vi "OpenVisualizations.vi"(8 "ErrorArray in":errorcluster[](array[cluster]), 11 "Visualization VI Paths":path[](array[path])) -> (0 "ErrorArray out":errorcluster[](array[cluster]))   [LabVIEW 2018]
uses:
  VisulaizationManagement/VisualizationManagerActions.ctl
  VisulaizationManagement/OpenVisualizationVIs.ctl
  <userlib>/NIST/NISTErrorLib/NISTErrorLib.lvlib
  NistPluggableModules/TestClass/Test.lvclass
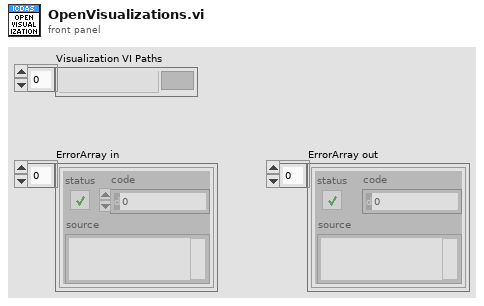
[diagram p1: front panel]
types:
  T1 = typedef "VisualizationManagerActions.ctl" = enum16{"Set", "LoadModVI", "PopOutModVI"}
  T2 = typedef "OpenVisualizationVIs.ctl" = cluster{"Module Name":string, "VI ref":refnum<vi>, "In SubPanel?":bool}
  T3 = typedef "cntlRefs.ctl" = cluster{"rngFGen":refnum<vi>, "rngDigitizer":refnum<vi>, "btnHide":refnum<vi>, "rngInst":refnum<vi>, "Instrument Modules":refnum<vi>, "RelativePathToINIFiles ":refnum<vi>, "PluginTree":refnum<vi>, "TestTree":refnum<vi>, "path.tstFile":refnum<vi>, "cmbxRunningModules":refnum<vi>, "TestDataSubPanel":refnum<vi>, "TestDataCaption":refnum<vi>, "btnPopInOut":refnum<vi>}
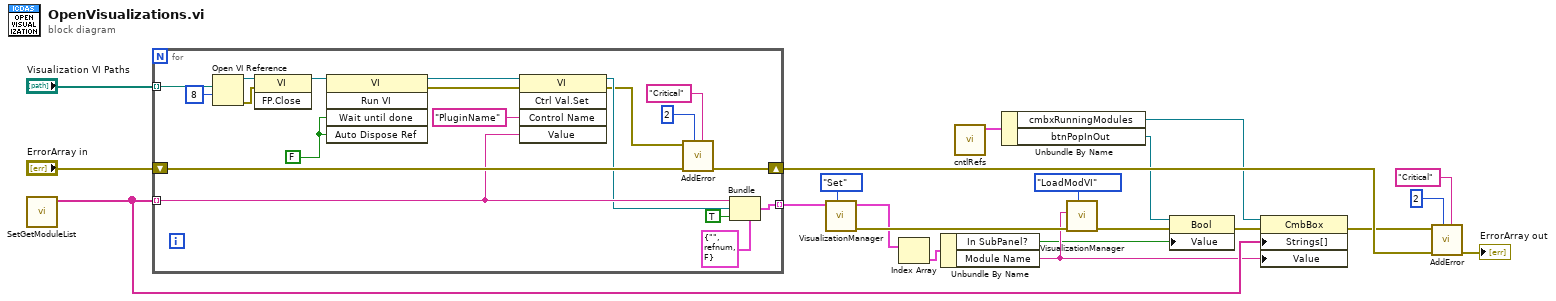
[diagram p0: block diagram]
diagram:
  n1 = call "SetGetModuleList.vi"() -> ("ModuleList"=w6:string[])  [unwired: 11 in]
  n2 = for {
    shift-right: [w33] -> w11
    shift-left: "ErrorArray in" -> [w34]
    tunnel: "Visualization VI Paths" -> [w30] mode=indexing
    tunnel: w6 -> [w27] mode=indexing
    tunnel: [w23] -> w17 mode=indexing
    w37 = FALSE ("Wait Until Done")
    n3 = Open VI Reference(vi path=w30, options=8) -> (vi reference=w35:refnum<vi>, error out=w39:errorcluster)  [unwired: 4 in]
    n4 = invoke class="VI" method="FP.Close"(reference=w35, error in=w39) -> (reference out=w36:refnum<vi>)  [unwired: 1 in, 2 out]
    n5 = invoke class="VI" method="Run VI"(reference=w36, "Wait until done"=w37, "Auto Dispose Ref"=w37) -> (reference out=w29:refnum<vi>, error out=w38:errorcluster)  [unwired: 2 in, 3 out]
    n6 = invoke class="VI" method="Ctrl Val.Set"(reference=w29, error in=w38, "Control Name"="PluginName", "Value"=w27) -> (reference out=w25:refnum<vi>, error out=w24:errorcluster)  [unwired: 1 in, 3 out]
    n7 = call <userlib>:"AddError.vi"("Severity"="Critical", "Priority"=u8 2, "ErrorArray In"=w34, "error in (no error)"=w24) -> ("ErrorArray Out"=w33:errorcluster[])  [unwired: 6 in, 1 out]
    n8 = Bundle(cluster=T2 {"Module Name"="", "VI ref"=refnum, "In SubPanel?"=FALSE} ("Open Visualization VIs"), "Module Name"=w27, "VI ref"=w25, "In SubPanel?"=TRUE) -> (w23:T2)
  }
  n9 = call "VisualizationManager.vi"("Action"=VisualizationManagerActions."Set", "Open Visualization VIs in"=w17) -> ("error out"=w18:errorcluster, "Open Visualization VIs out"=w16:T2[])  [unwired: 8 in]
  n10 = Index Array(array=w16) -> (element=w19:T2)  [unwired: 1 in]
  n11 = Unbundle By Name(w19) -> ("In SubPanel?"=w1:bool, "Module Name"=w4:string)
  n12 = call "cntlRefs.vi"() -> ("cntlRefs"=w9:T3)  [unwired: 10 in, 1 out]
  n13 = Unbundle By Name(w9) -> ("cmbxRunningModules"=w7:refnum<vi>, "btnPopInOut"=w2:refnum<vi>)
  n14 = call "VisualizationManager.vi"("Action"=VisualizationManagerActions."LoadModVI", "error in (no error)"=w18, "Module Name"=w4) -> ("error out"=w12:errorcluster)  [unwired: 7 in, 1 out]
  n15 = property class="Bool"(reference=w2, error in=w12, "Value"=w1) -> (error out=w3:errorcluster)  [unwired: 1 out]
  n16 = property class="CmbBox"(reference=w7, error in=w3, "Strings[]"=w6, "Value"=w4) -> (error out=w8:errorcluster)  [unwired: 1 out]
  n17 = call <userlib>:"AddError.vi"("Severity"="Critical", "Priority"=u8 2, "ErrorArray In"=w11, "error in (no error)"=w8) -> ("ErrorArray Out"=→"ErrorArray out":errorcluster[])  [unwired: 6 in, 1 out]
